vi "DB - [Config].[StationSysRelation].vi"(6 "[ClientName]":string="F001", 7 "DB Connection":T2={"Open"=TRUE, "Close"=TRUE}, 8 "error in (no error)":errorcluster, 9 "[StationId]":string="F001", 10 "[PlantId]":string="4070", 11 "connection reference":T1) -> (0 "SUMMARY":errorcluster, 2 "[SystemId]":string, 3 "connection reference":T1)   [LabVIEW 2013]
uses:
  <vilib>/addons/database/Connection.llb/Conn ObjectReference.ctl
  Controls/DB - OpenClose.ctl
  <vilib>/addons/database/Connection.llb/Conn Execute.vi
  <vilib>/addons/database/Recordset.llb/Rec Fetch Recordset Data (R).vi
  <vilib>/addons/database/Recordset.llb/Rec Destroy - Connection.vi
  Controls/Global SRTRS.vi
  <vilib>/addons/database/Connection.llb/DB Tools Open Connec (String).vi
  <vilib>/addons/database/_DB Variant To Data/Database Variant To Data.xnode
  <vilib>/addons/database/NI_Database_API.lvlib
panel:
  out "Close":errorcluster
  in  "DB.Schema.Table \nSRTRS.Config.System":string="SRTRS.Config.System"
  out "SQL Statement":string
  out "data":string[][](array[string])
  in  "DB.Schema.Table \nSRTRS.Config.StationSysRelation":string="SRTRS.Config.StationSysRelation"
  in  "DB.Schema.Table\nSRTRS.Config.Station":string="SRTRS.Config.Station"
  out "Connection Information":T3={"Connection "="SQL Server 32bit HPEnvy", "Username"="admin", "Password"="admin123"}
  # "2014-11-07 10:06\n[StationId]                        [Station Description]                        [SystemId]                      [System Description]"
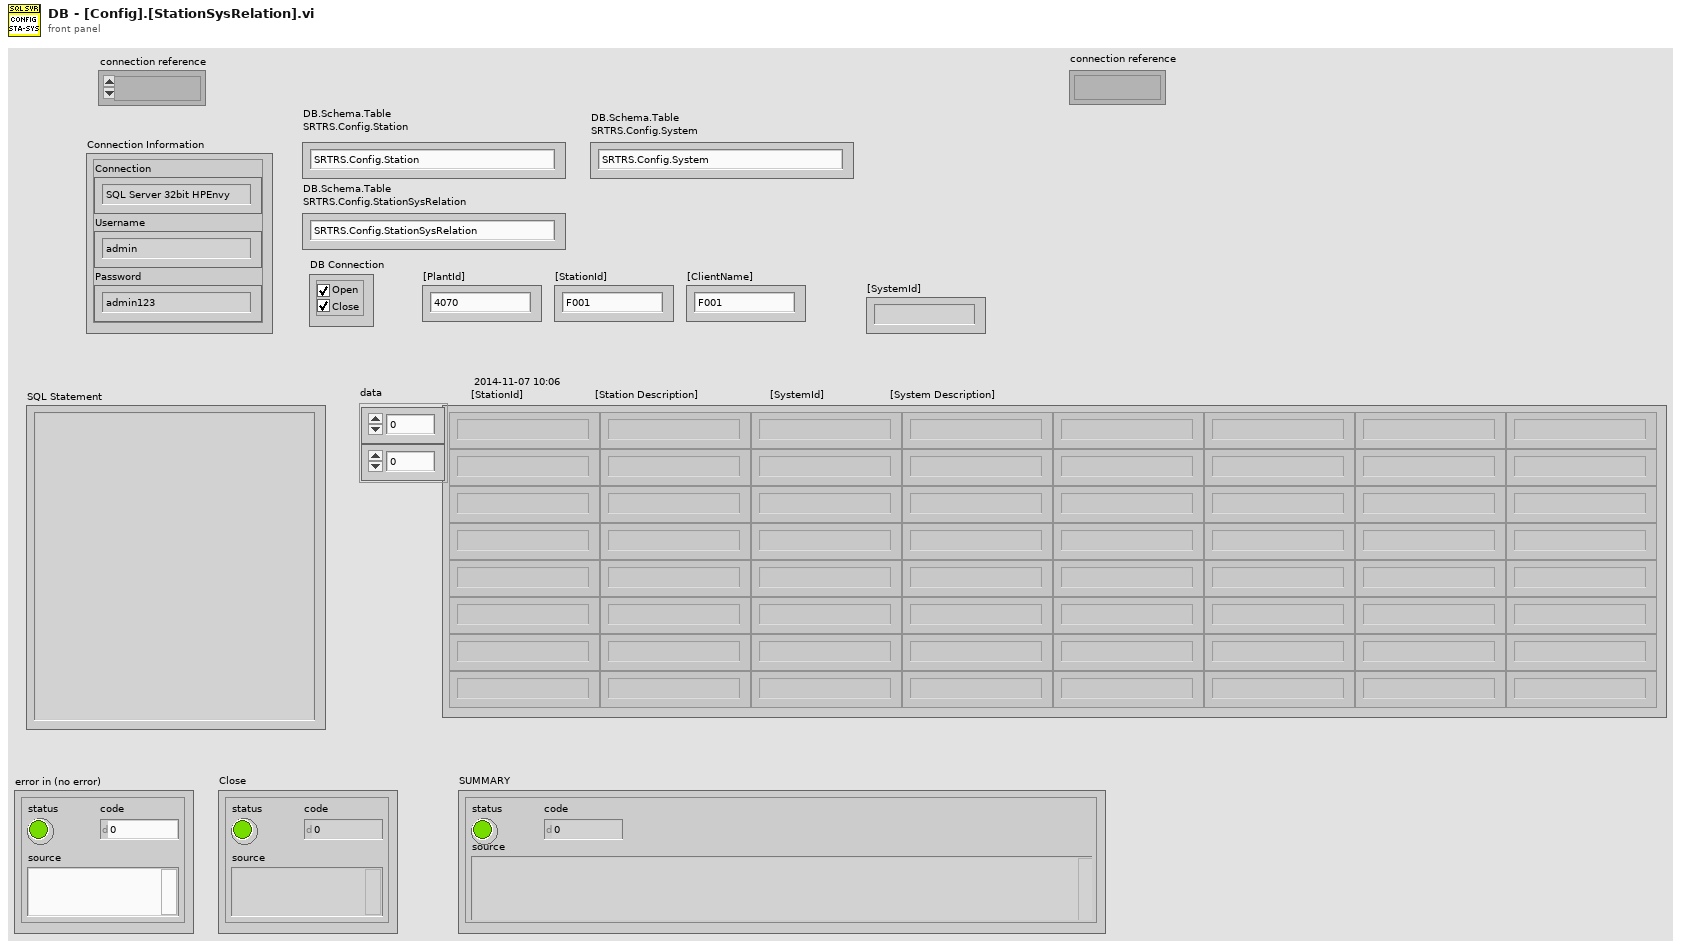
[diagram p1: front panel]
types:
  T1 = typedef "NI_Database_API.lvlib/Conn ObjectReference.ctl" = refnum<k1>
  T2 = typedef "DB - OpenClose.ctl" = cluster{"Open":bool, "Close":bool}
  T3 = cluster{"Connection ":string, "Username":string, "Password":string}
  T4 = typedef "Enum - InteractiveMode-SubVIMode.ctl" = enum16{"Interactive", "subVI Mode"}
  T5 = typedef "DB - DB.Schema.Table.ctl" = cluster{"DB":string, "Schema":string, "Table":string}
  T6 = typedef "Connection Information Cluster.ctl" = cluster{"Connection ":string, "Username":string, "Password":string}
  T7 = typedef "NI_Database_API.lvlib/Rec ObjectReference.ctl" = refnum<k1>
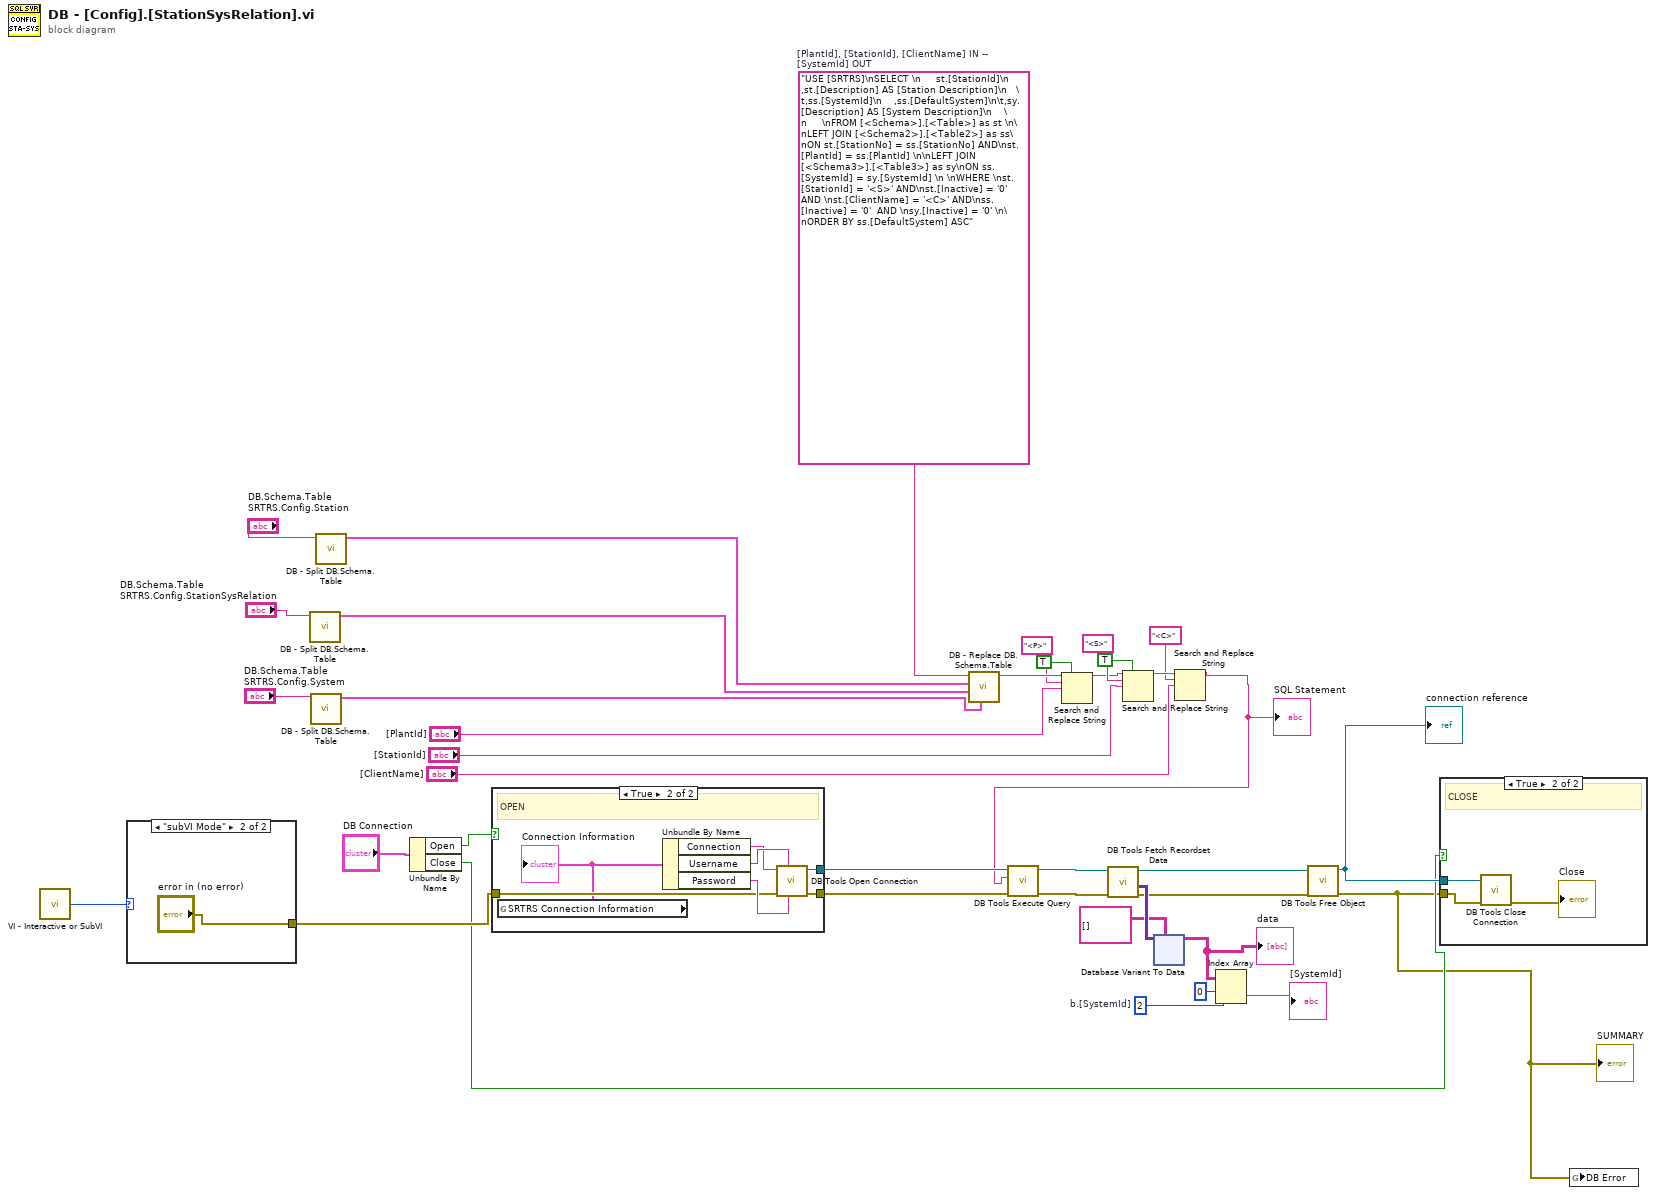
[diagram p0: block diagram]
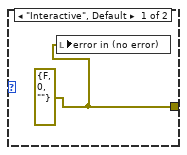
[diagram p3: hidden frame]
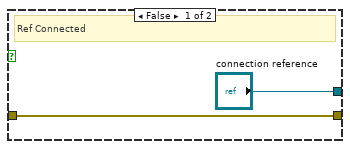
[diagram p4: hidden frame]
diagram:
  w6 = 2  # b.[SystemId]
  w9 = "USE [SRTRS]\nSELECT \n     st.[StationId]\n    ,st.[Description] AS [Station Description]\n   \t,ss.[SystemId]\n    ,ss.[DefaultSystem]\n\t,sy.[Description] AS [System Description]\n    \n     \nFROM [<Schema>].[<Table>] as st \n\nLEFT JOIN [<Schema2>].[<Table2>] as ss\nON st.[StationNo] = ss.[StationNo] AND\nst.[PlantId] = ss.[PlantId] \n\nLEFT JOIN [<Schema3>].[<Table3>] as sy\nON ss.[SystemId] = sy.[SystemId] \n \nWHERE \nst.[StationId] = '<S>' AND\nst.[Inactive] = '0' AND \nst.[ClientName] = '<C>' AND\nss.[Inactive] = '0'  AND \nsy.[Inactive] = '0' \n\nORDER BY ss.[DefaultSystem] ASC"  # [PlantId], [StationId], [ClientName] IN --  [SystemId] OUT
  n1 = call "VI - Interactive or SubVI.vi"() -> ("Mode"=w36:T4)  [unwired: 5 in]
  n2 = case shown="\"subVI Mode\"" w36 {
    tunnel: [w39 "error in (no error)"] -> w35
    frame "Interactive", Default {
      w39 = errorcluster {"status"=FALSE, "code"=0, "source"=""} ("error in (no error)")
      n3 = local write "error in (no error)"(w39) -> ()
    }
    frame "subVI Mode" {
    }
  }
  n4 = call "DB - Split DB.Schema.Table.vi"("DB.Schema.Table"="DB.Schema.Table \nSRTRS.Config.StationSysRelation") -> ("DB.Schema.Table"=w18:T5)  [unwired: 10 in]
  n5 = call "DB - Split DB.Schema.Table.vi"("DB.Schema.Table"="DB.Schema.Table \nSRTRS.Config.System") -> ("DB.Schema.Table"=w16:T5)  [unwired: 10 in]
  n6 = call "DB - Split DB.Schema.Table.vi"("DB.Schema.Table"="DB.Schema.Table\nSRTRS.Config.Station") -> ("DB.Schema.Table"=w22:T5)  [unwired: 10 in]
  n7 = Unbundle By Name("DB Connection") -> ("Open"=w37:bool, "Close"=w25:bool)
  n8 = case shown="True" w37 {
    tunnel: ["connection reference" w46] -> w28
    tunnel: w35 -> [w41 w45]
    tunnel: [w41 w44] -> w27
    frame False {
      # "Ref Connected"
    }
    frame True {
      # "OPEN"
      n9 = global read "Global SRTRS.vi" "SRTRS Connection Information"() -> (w43:T6)
      "Connection Information" <- w43
      n10 = Unbundle By Name(w43) -> ("Connection"=w48:string, "Username"=w49:string, "Password"=w47:string)
      n11 = call-poly <vilib>:"DB Tools Open Connection.vi"("password"=w47, "userID"=w49, "error in (no error)"=w45, "connection information"=w48) -> ("error out"=w44:errorcluster, "connection reference"=w46:T1)  [unwired: 4 in]
    }
  }
  n12 = call "DB - Replace DB.Schema.Table.vi"("DB.Schema.Table 3"=w16, "DB.Schema.Table 2"=w18, "DB.Schema.Table"=w22, "string in"=w9) -> ("string out"=w21:string)  [unwired: 6 in, 1 out]
  n13 = Search and Replace String(replace all?=TRUE ("replace all? (F)"), input string=w21, search string="<P>", replace string="[PlantId]") -> (result string=w11:string)  [unwired: 4 in, 3 out]
  n14 = Search and Replace String(replace all?=TRUE ("replace all? (F)"), input string=w11, search string="<S>", replace string="[StationId]") -> (result string=w4:string)  [unwired: 4 in, 3 out]
  n15 = Search and Replace String(input string=w4, search string="<C>", replace string="[ClientName]") -> (result string=w3:string)  [unwired: 5 in, 3 out]
  "SQL Statement" <- w3
  n16 = call-poly <vilib>:"DB Tools Execute Query.vi"("error in (no error)"=w27, "SQL query"=w3, "connection reference"=w28) -> ("error out"=w34:errorcluster, "recordset reference"=w33:T7)  [unwired: 5 in]
  n17 = call-poly <vilib>:"DB Tools Fetch Recordset Data.vi"("error in (no error)"=w34, "recordset reference"=w33) -> ("error out"=w29:errorcluster, "recordset data"=w32:variant[][], "recordset reference out"=w30:T7)  [unwired: 3 in]
  n18 = xnode "Database Variant To Data"("database variant"=w32, "type"=string[][] []) -> ("data"=w8:string[][])  [unwired: 1 in, 1 out]
  "data" <- w8
  n19 = Index Array(array=w8, index (row)=0, index (col)=w6) -> (element=→"[SystemId]":string)
  n20 = call-poly <vilib>:"DB Tools Free Object.vi"("error in (no error)"=w29, "recordset reference"=w30) -> ("error out"=w15:errorcluster, "connection reference"=w26:T1)  [unwired: 8 in]
  "SUMMARY" <- w15
  "connection reference" <- w26
  n21 = case shown="True" w25 {
    tunnel: w26 -> [_ w52]
    tunnel: w15 -> [_ w51]
    frame False {
      # "Ref Connected"
    }
    frame True {
      # "CLOSE"
      n22 = call <vilib>:"DB Tools Close Connection.vi"("error in (no error)"=w51, "connection reference"=w52) -> ("error out"=→"Close":errorcluster)  [unwired: 5 in]
    }
  }
  n23 = global write "Global SRTRS.vi" "DB Error"(w15) -> ()
